vi "Label Array to Label String.vi"(1 "Label Array":i16[](array[numeric])) -> (0 "Label String":string)   [LabVIEW 2010]
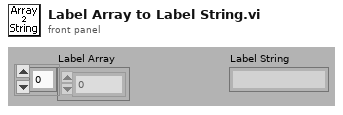
[diagram p1: front panel]
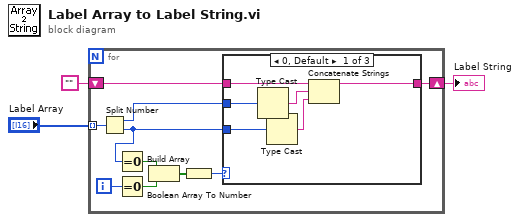
[diagram p0: block diagram]
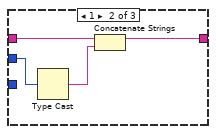
[diagram p2: hidden frame]
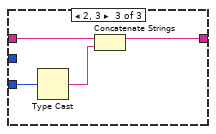
[diagram p3: hidden frame]
diagram:
  n1 = for {
    shift-right: [w12] -> w1
    shift-left: "" -> [w13]
    tunnel: "Label Array" -> [w11] mode=indexing
    i -> [w9]
    n2 = Split Number(x=w11) -> (hi(x)=w10:u8, lo(x)=w8:u8)
    n3 = Equal To 0?(x=w8) -> (x = 0?=w7:bool)
    n4 = Equal To 0?(x=w9) -> (x = 0?=w6:bool)
    n5 = Build Array(w7, w6) -> (w5:bool[])
    n6 = Boolean Array To Number(Boolean array=w5) -> (number=w4:u32)
    n7 = case shown="0, Default" w4 {
      tunnel: w13 -> [w19 w23 w27]
      tunnel: [w16 w21 w25] -> w12
      tunnel: w8 -> [w14 _ w24]
      tunnel: w10 -> [w15 w20 _]
      frame 0, Default {
        n8 = Type Cast(x=w15) -> (*(type *) &x=w18:string)  [unwired: 1 out]
        n9 = Type Cast(x=w14) -> (*(type *) &x=w17:string)  [unwired: 1 out]
        n10 = Concatenate Strings(w19, w18, w17) -> (w16:string)
      }
      frame 1 {
        n11 = Type Cast(x=w20) -> (*(type *) &x=w22:string)  [unwired: 1 out]
        n12 = Concatenate Strings(w23, w22) -> (w21:string)
      }
      frame 2, 3 {
        n13 = Type Cast(x=w24) -> (*(type *) &x=w26:string)  [unwired: 1 out]
        n14 = Concatenate Strings(w27, w26) -> (w25:string)
      }
    }
  }
  "Label String" <- w1
